vi "ConvertBARInputBytes.vi"(11 "BAR Bytes":u8[](array[numeric])) -> (3 "Pressure (Torr)":sgl)   [LabVIEW 2011]
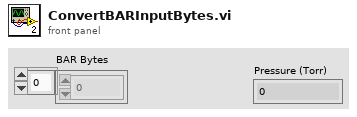
[diagram p1: front panel]
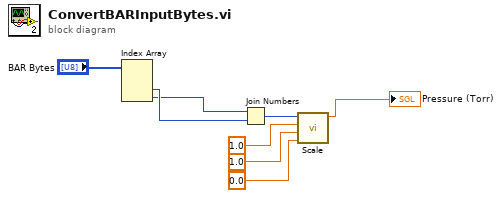
[diagram p0: block diagram]
diagram:
  n1 = Index Array(array="BAR Bytes") -> (element #2=w7:u8, element #3=w6:u8)  [unwired: 3 in, 1 out]
  n2 = Join Numbers(hi=w6, lo=w7) -> ((hi.lo)=w5:u16)
  n3 = call "Scale.vi"("Offset"=0.0, "Factor"=1.0, "FullScale"=1.0, "Input"=w5) -> ("Output"=→"Pressure (Torr)":dbl)  [unwired: 7 in]
